vi "GetPortString.vi"(0 "nDeviceNo":u32) -> (4 "ExternOut1":string, 6 "ExternOut2":string, 8 "ExternOut3":string, 10 "ExternOut4":string, 12 "ExternIn1":string, 13 "ExternIn2":string, 14 "ExternIn3":string)   [LabVIEW 2015]
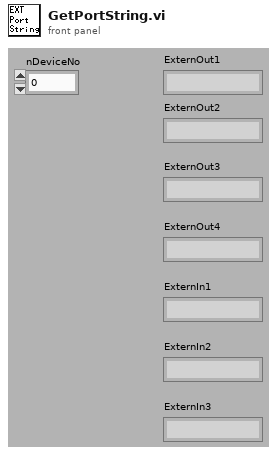
[diagram p1: front panel]
types:
  T1 = cluster{"ReturnValue":u32, "ErrorCode":u32, "error ":errorcluster}
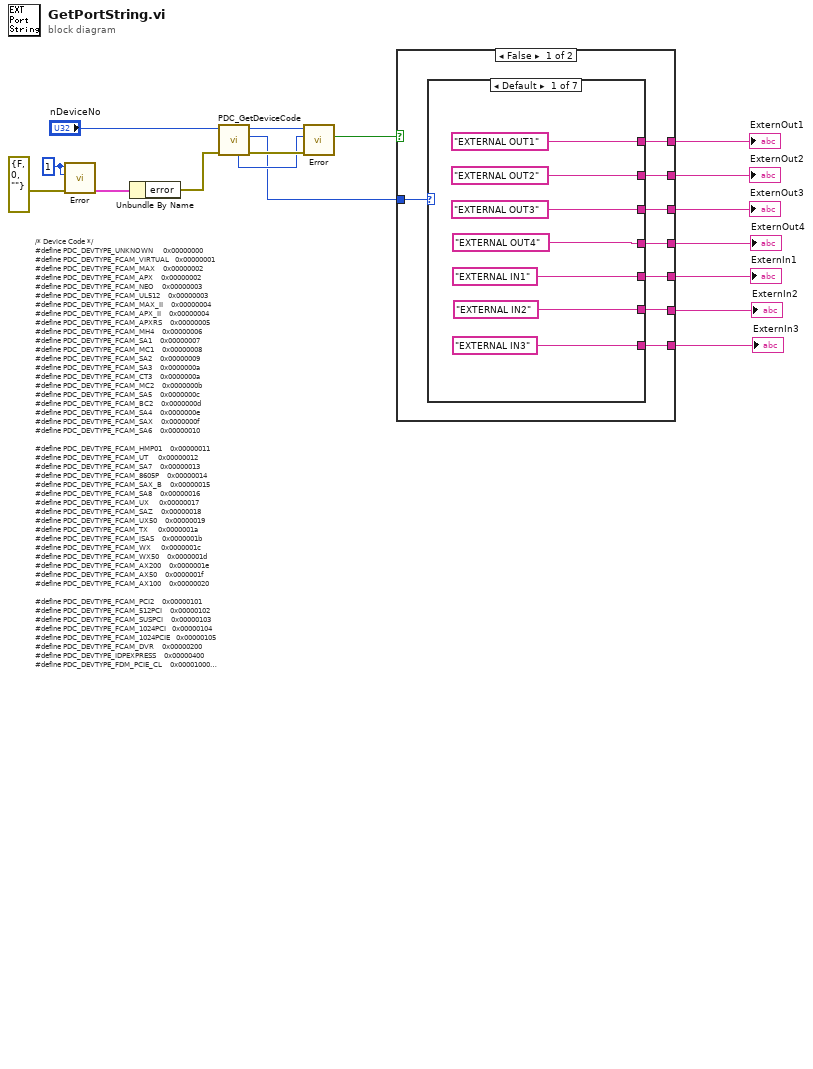
[diagram p0: block diagram]
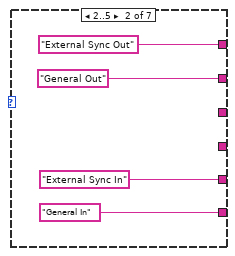
[diagram p2: hidden frame]
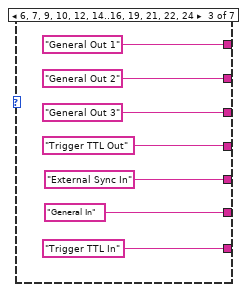
[diagram p3: hidden frame]
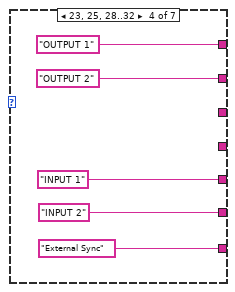
[diagram p4: hidden frame]
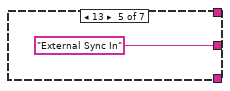
[diagram p5: hidden frame]
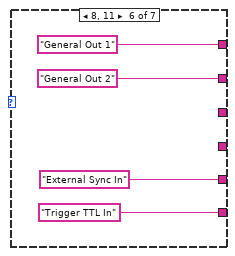
[diagram p6: hidden frame]
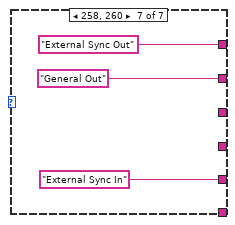
[diagram p7: hidden frame]
diagram:
  w17 = u32 1 ("return type")
  # "/*\tDevice Code\t*/\n#define\tPDC_DEVTYPE_UNKNOWN\t\t\t\t\t0x00000000\n#define\tPDC_DEVTYPE_FCAM_VIRTUAL\t\t\t0x00000001\n#define\tPDC_DEVTYPE_FCAM_MAX\t\t\t\t0x00000002\n#define\tPDC_DEVTYPE_FCAM_APX\t\t\t\t0x00000002\n#define\tPDC_DEVTYPE_FCAM_NEO\t\t\t\t0x00000003\n#define\tPDC_DEVTYPE_FCAM_UL512\t\t\t\t0x00000003\n#define\tPDC_DEVTYPE_FCAM_MAX_II\t\t\t\t0x00000004\n#define\tPDC_DEVTYPE_FCAM_APX_II\t\t\t\t0x00000004\n#define\tPDC_DEVTYPE_FCAM_APXRS\t\t\t\t0x00000005\n#define\tPDC_DEVTYPE_FCAM_MH4\t\t\t\t0x00000006\n#define\tPDC_DEVTYPE_FCAM_SA1\t\t\t\t0x00000007\n#define\tPDC_DEVTYPE_FCAM_MC1\t\t\t\t0x00000008\n#define\tPDC_DEVTYPE_FCAM_SA2\t\t\t\t0x00000009\n#define\tPDC_DEVTYPE_FCAM_SA3\t\t\t\t0x0000000a\n#define\tPDC_DEVTYPE_FCAM_CT3\t\t\t\t0x0000000a\n#define\tPDC_DEVTYPE_FCAM_MC2\t\t\t\t0x0000000b\n#define\tPDC_DEVTYPE_FCAM_SA5\t\t\t\t0x0000000c\n#define\tPDC_DEVTYPE_FCAM_BC2\t\t\t\t0x0000000d\n#define\tPDC_DEVTYPE_FCAM_SA4\t\t\t\t0x0000000e\n#define\tPDC_DEVTYPE_FCAM_SAX\t\t\t\t0x0000000f\n#define\tPDC_DEVTYPE_FCAM_SA6\t\t\t\t0x00000010\n\n#define\tPDC_DEVTYPE_FCAM_HMP01\t\t\t\t0x00000011\n#define PDC_DEVTYPE_FCAM_UT\t\t\t\t\t0x00000012\n#define PDC_DEVTYPE_FCAM_SA7\t\t\t\t0x00000013\n#define PDC_DEVTYPE_FCAM_8605P\t\t\t\t0x00000014\n#define\tPDC_DEVTYPE_FCAM_SAX_B\t\t\t\t0x00000015\n#define\tPDC_DEVTYPE_FCAM_SA8\t\t\t\t0x00000016\n#define\tPDC_DEVTYPE_FCAM_UX\t\t\t\t\t0x00000017\n#define\tPDC_DEVTYPE_FCAM_SAZ\t\t\t\t0x00000018\n#define\tPDC_DEVTYPE_FCAM_UX50\t\t\t\t0x00000019\n#define\tPDC_DEVTYPE_FCAM_TX\t\t\t\t\t0x0000001a\n#define\tPDC_DEVTYPE_FCAM_ISAS\t\t\t\t0x0000001b\n#define PDC_DEVTYPE_FCAM_WX\t\t\t\t\t0x0000001c\n#define PDC_DEVTYPE_FCAM_WX50\t\t\t\t0x0000001d\n#define PDC_DEVTYPE_FCAM_AX200\t\t\t\t0x0000001e\n#define PDC_DEVTYPE_FCAM_AX50\t\t\t\t0x0000001f\n#define PDC_DEVTYPE_FCAM_AX100\t\t\t\t0x00000020\n\n#define\tPDC_DEVTYPE_FCAM_PCI2\t\t\t\t0x00000101\n#define\tPDC_DEVTYPE_FCAM_512PCI\t\t\t\t0x00000102\n#define\tPDC_DEVTYPE_FCAM_SUSPCI\t\t\t\t0x00000103\n#define\tPDC_DEVTYPE_FCAM_1024PCI\t\t\t0x00000104\n#define\tPDC_DEVTYPE_FCAM_1024PCIE\t\t\t0x00000105\n#define PDC_DEVTYPE_FCAM_DVR\t\t\t\t0x00000200\n#define\tPDC_DEVTYPE_IDPEXPRESS\t\t\t\t0x00000400\n#define\tPDC_DEVTYPE_FDM_PCIE_CL\t\t\t\t0x00001000\n#define\tPDC_DEVTYPE_FCAM_SP8\t\t\t\t0x00010000\n#define\tPDC_DEVTYPE_PCAM_SPEEDER\t\t\t0x00100000\n#define\tPDC_DEVTYPE_PCAM_SPEEDER_V2\t\t\t0x00100001\n#define\tPDC_DEVTYPE_PI5\t\t\t\t\t\t0x00000410"
  n1 = call "Error.vi"("error in (no error)"=errorcluster {"status"=FALSE, "code"=0, "source"=""}, "ErrorCode"=w17, "ReturnValue"=w17) -> ("Error_Out"=w15:T1)  [unwired: 8 out]
  n2 = Unbundle By Name(w15) -> ("error"=w14:errorcluster)
  n3 = call "PDC_GetDeviceCode.vi"("error in (no error)"=w14, "DeviceNo"="nDeviceNo") -> ("error out"=w13:errorcluster, "ID"=w9:u32, "ReturnValue"=w12:u32, "ErrorCode"=w11:u32)  [unwired: 6 out]
  n4 = call "Error.vi"("error in (no error)"=w13, "ErrorCode"=w11, "ReturnValue"=w12) -> ("Error?"=w10:bool)  [unwired: 8 out]
  n5 = case shown="False" w10 {
    tunnel: w9 -> [w25 _]
    tunnel: [w24 _] -> w7
    tunnel: [w23 _] -> w6
    tunnel: [w22 _] -> w5
    tunnel: [w21 _] -> w4
    tunnel: [w20 _] -> w3
    tunnel: [w19 _] -> w2
    tunnel: [w18 _] -> w1
    frame False {
      n6 = case shown="Default" w25 {
        tunnel: ["EXTERNAL OUT1" "External Sync Out" "General Out 1" "OUTPUT 1" _ "General Out 1" "External Sync Out"] -> w24
        tunnel: ["EXTERNAL OUT2" "General Out" "General Out 2" "OUTPUT 2" _ "General Out 2" "General Out"] -> w23
        tunnel: ["EXTERNAL OUT3" _ "General Out 3" _ _ _ _] -> w22
        tunnel: ["EXTERNAL OUT4" _ "Trigger TTL Out" _ _ _ _] -> w21
        tunnel: ["EXTERNAL IN1" "External Sync In" "External Sync In" "INPUT 1" "External Sync In" "External Sync In" "External Sync In"] -> w20
        tunnel: ["EXTERNAL IN2" "General In" "General In" "INPUT 2" _ "Trigger TTL In" _] -> w19
        tunnel: ["EXTERNAL IN3" _ "Trigger TTL In" "External Sync" _ _ _] -> w18
        frame Default {
        }
        frame 2..5 {
        }
        frame 6, 7, 9, 10, 12, 14..16, 19, 21, 22, 24 {
        }
        frame 23, 25, 28..32 {
        }
        frame 13 {
        }
        frame 8, 11 {
        }
        frame 258, 260 {
        }
      }
    }
    frame True {
    }
  }
  "ExternOut1" <- w7
  "ExternOut2" <- w6
  "ExternOut3" <- w5
  "ExternOut4" <- w4
  "ExternIn1" <- w3
  "ExternIn2" <- w2
  "ExternIn3" <- w1
